vi "files_in_folder.vi"(11 "folder path":path) -> (3 "Array":path[](array[path]))   [LabVIEW 2017]
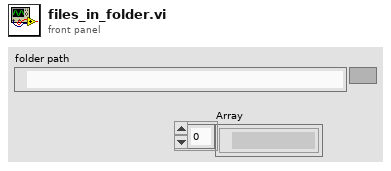
[diagram p1: front panel]
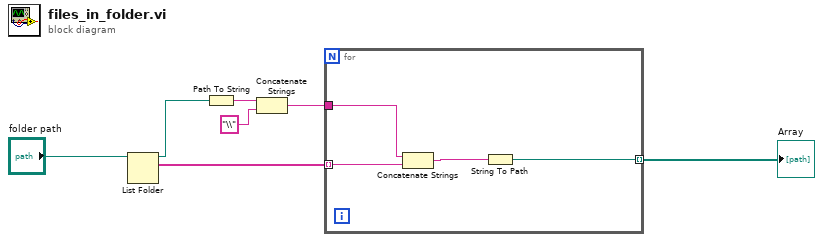
[diagram p0: block diagram]
diagram:
  n1 = List Folder(path="folder path") -> (path out=w2:path, filenames=w6:string[])  [unwired: 3 in, 2 out]
  n2 = Path To String(path=w2) -> (string=w3:string)
  n3 = Concatenate Strings(w3, "\\" ("string")) -> (w1:string)
  n4 = for {
    tunnel: w6 -> [w11] mode=indexing
    tunnel: [w9] -> w7 mode=indexing
    tunnel: w1 -> [w8]
    n5 = Concatenate Strings(w8, w11) -> (w10:string)
    n6 = String To Path(string=w10) -> (path=w9:path)
  }
  "Array" <- w7
